vi "Vision Research Phantom Series PhCon PhNVMErase.vi"(0 "CN in":u32=1, 5 "Error In (no error)":errorcluster, 7 "CallID":u32) -> (14 "CN out":u32=1, 19 "Error Out":errorcluster)   [LabVIEW 2013, in "VRI.lvlib"]
doc: "PhCon.dll\n\nPhNVMErase\nHRESULT PhNVMErase (UINT CN, UINT CallID);\n\nParameters Description\nCN (in) Camera number.\nCallID (in) Choose a CallID(unsigned int <= 15) and pass it \n in the place of the Function pointer parameter. \n To retrieve progress information for that call, \n you must call LVProgress with chosen CallID \n within a loop. The time consuming call and the \n LVProgress call must be in separate threads.\nReturn HRESULT (0=Ok)\nComments Erase all the cines from NVM\n\nWritten by:\nBLOOMY CONTROLS, INC\nWINDSOR, CT 06095, USA\n860-298-9925\nwww.bloomy.com\nV1.0.0\nMay, 2004"
uses:
  VRI.lvlib
  Phantom DLLs/PhCon.dll
panel:
  # "For instructions on the use of this VI, press Ctrl+H to display the help window and move the mouse over the icon, controls, and indicators"
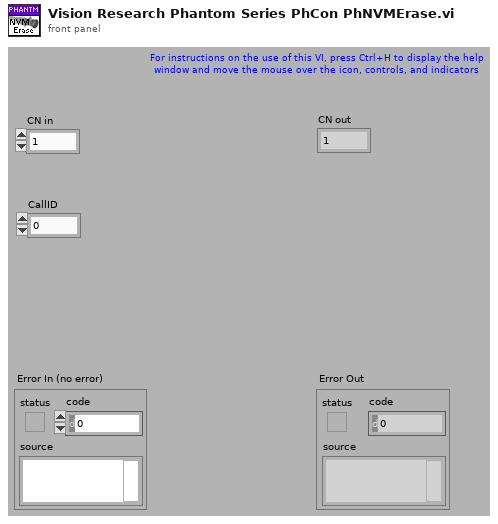
[diagram p1: front panel]
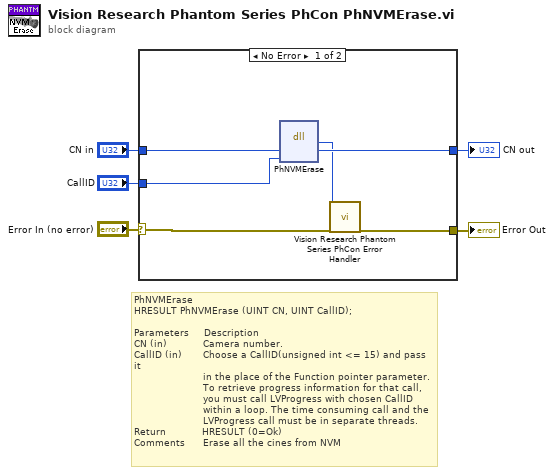
[diagram p0: block diagram]
diagram:
  # "PhNVMErase\nHRESULT PhNVMErase (UINT CN, UINT CallID);\n\nParameters     Description\nCN (in)            Camera number.\nCallID (in)       Choose a CallID(unsigned int <= 15) and pass it \n                       in the place of the Function pointer parameter. \n                       To retrieve progress information for that call, \n                       you must call LVProgress with chosen CallID \n                       within a loop. The time consuming call and the \n                       LVProgress call must be in separate threads.\nReturn            HRESULT (0=Ok)\nComments      Erase all the cines from NVM"
  n1 = case shown="No Error" "Error In (no error)" {
    selector: "Error In (no error)" -> [w11 w12]
    tunnel: [w10 w12] -> w4
    tunnel: "CN in" -> [w9 _]
    tunnel: [w8 _] -> w2
    tunnel: "CallID" -> [w7 _]
    frame No Error {
      n2 = dll-call lib="C:/Projects/SDK/32-bit/Vision Research Phantom Series Labview Driver/Phantom DLLs/PhCon.dll" fn="PhNVMErase"("CN"=w9, "CallID"=w7) -> ("HRESULT"=w6:i32, "CN"=w8:u32)  [unwired: 4 in, 2 out]
      n3 = call "Vision Research Phantom Series PhCon Error Handler.vi"("ErrNo"=w6, "Error In (no error)"=w11) -> ("Error Out"=w10:errorcluster)  [unwired: 17 out]
    }
    frame Error {
    }
  }
  "Error Out" <- w4
  "CN out" <- w2
